vi "Get Test Limits Source File Name.vi"(8 "error in (no error)":errorcluster, 11 "Test Limits File Path":path) -> (0 "error out":errorcluster, 3 "Source File":string)   [LabVIEW 2025, in "Test Limits.lvlib"]
uses:
  Test Limits.lvlib
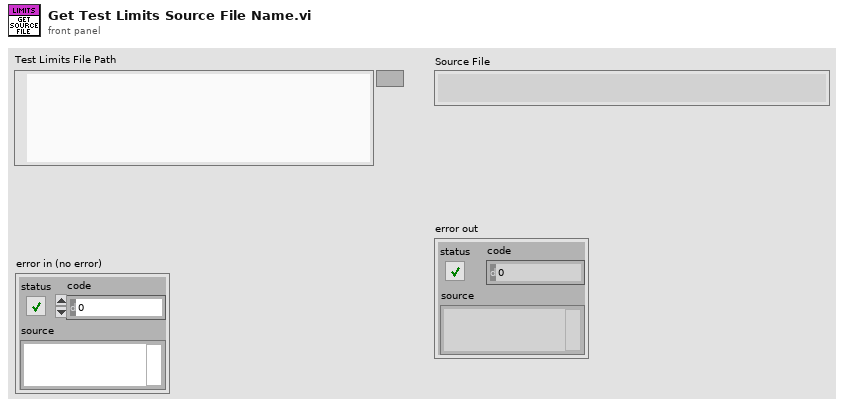
[diagram p1: front panel]
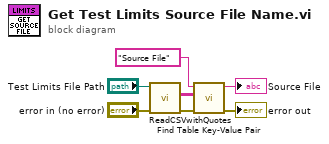
[diagram p0: block diagram]
diagram:
  n1 = call "ReadCSVwithQuotes.vi"("error in (no error)"="error in (no error)", "File Path"="Test Limits File Path") -> ("error out"=w3:errorcluster, "Array"=w4:string[][])  [unwired: 7 in, 1 out]
  n2 = call "Find Table Key-Value Pair.vi"("error in (no error)"=w3, "Table Array"=w4, "Key Regex"="Source File") -> ("error out"=→"error out":errorcluster, "Value"=→"Source File":string)  [unwired: 7 in]
